vi "NormaliseProfile.vi"(5 "ResampleHeights":dbl[](array[numeric])=[25.4, 38.1, 50.8, 76.2, 101.6, 127.0, 152.4, 203.2, 254.0, 304.8, 406.4, 508.0, 609.6, 812.8, 1219.2, 1524.0], 6 "Zref":dbl=508.0 min=0.0, 7 "ResampleToN":i32, 10 "zUClusterIn":cluster{dbl[], dbl[]}, 11 "Resampler":T1) -> (1 "U(Zref)":dbl, 2 "zUClusterNormalised":cluster{dbl[], dbl[]}, 3 "zUClusterNormalisedResampled":cluster{dbl[], dbl[]})   [LabVIEW 2014]
uses:
  Resampler.ctl
  <vilib>/Analysis/NI_AALPro.lvlib
  <vilib>/gmath/NI_Gmath.lvlib
panel:
  in  "Interpolation":i32(ring)=1 items=["nearest", "linear", "spline", "cubic Hermite", "Lagrange"]
  in  "binTolerance":dbl=10.0
  out "firstBelow":dbl
  out "firstAbove":dbl
  out "XY Graph":cluster{dbl[], dbl[]}[](graph)
  # "Fit using values at  measurement Z heights"
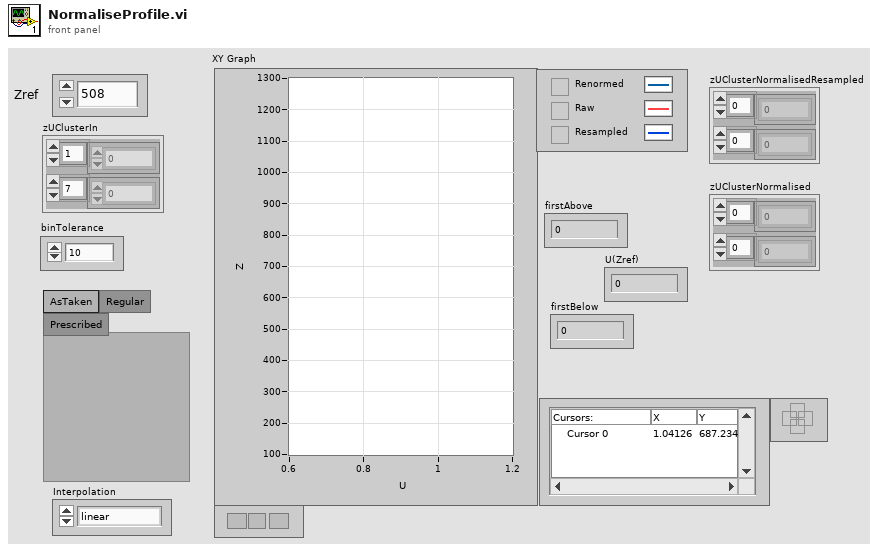
[diagram p1: front panel]
types:
  T1 = typedef "Resampler.ctl" = enum32{"AsTaken", "Regular", "Prescribed"}
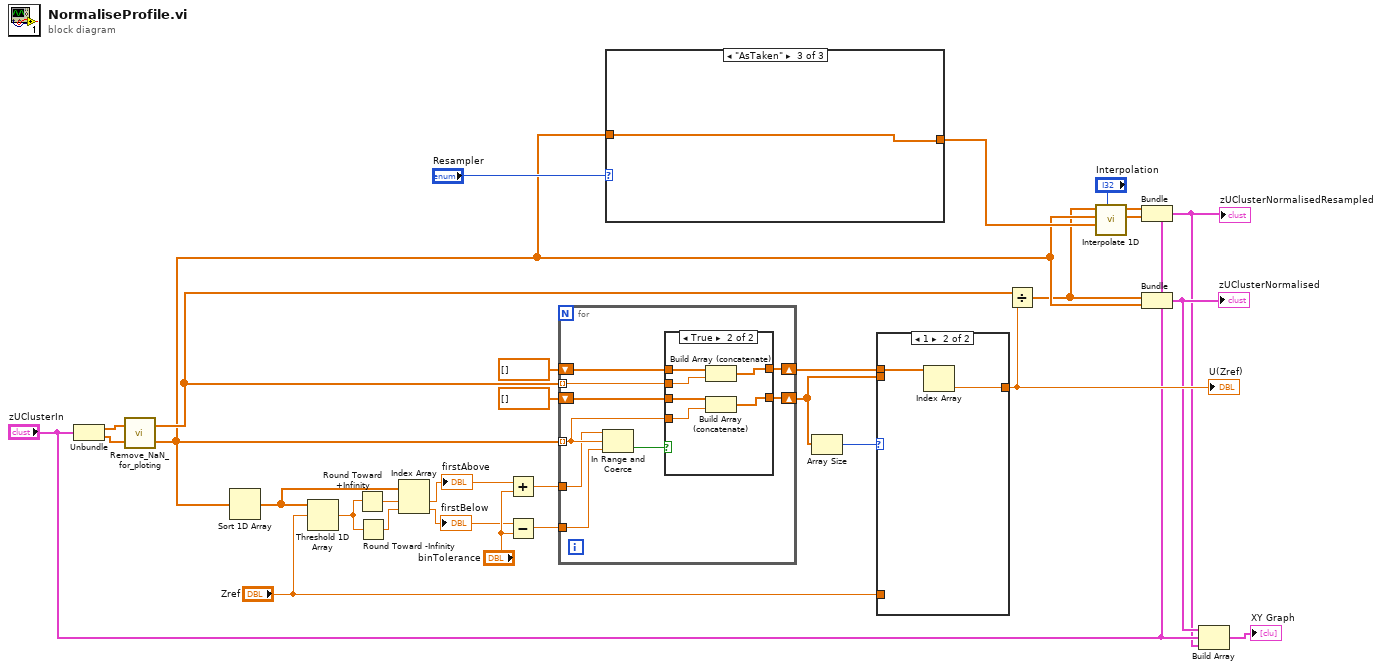
[diagram p0: block diagram]
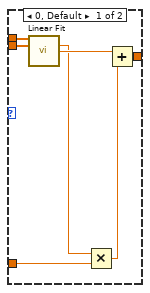
[diagram p2: hidden frame]
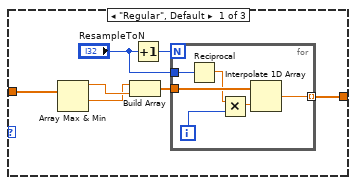
[diagram p3: hidden frame]
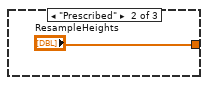
[diagram p4: hidden frame]
diagram:
  n1 = Unbundle("zUClusterIn") -> (w15:dbl[], w16:dbl[])
  n2 = call "Remove_NaN_for_ploting.vi"("Array 2"=w16, "Array 1"=w15) -> ("Array 2 Out"=w6:dbl[], "Array 1 Out"=w14:dbl[])
  n3 = Sort 1D Array(array=w6) -> (sorted array=w29:dbl[])
  n4 = Threshold 1D Array(2:"Zref", 3:w29) -> (0:w30:dbl)  [unwired: 1 in]
  n5 = Round Toward +Infinity(x=w30) -> (ceil(x): smallest int >= x=w28:dbl)
  n6 = Round Toward -Infinity(1:w30) -> (0:w27:dbl)
  n7 = Index Array(array=w29, index #1=w28, index #2=w27) -> (element #1=w4:dbl, element #2=w3:dbl)
  "firstAbove" <- w4
  "firstBelow" <- w3
  n8 = Add(x=w4, y="binTolerance") -> (x+y=w25:dbl)
  n9 = Subtract(x=w3, y="binTolerance") -> (x-y=w24:dbl)
  n10 = for {
    tunnel: w14 -> [w38] mode=indexing
    tunnel: w6 -> [w39] mode=indexing
    tunnel: w25 -> [w33]
    tunnel: w24 -> [w32]
    shift-right: [w37] -> w23
    shift-left: dbl[] [] -> [w36]
    shift-right: [w34] -> w2
    shift-left: dbl[] [] -> [w35]
    n11 = In Range and Coerce(upper limit=w33, x=w39, lower limit=w32) -> (In Range?=w31:bool)  [unwired: 1 out]
    n12 = case shown="True" w31 {
      tunnel: w39 -> [_ w47]
      tunnel: w38 -> [_ w46]
      tunnel: [w41 w45] -> w37
      tunnel: w36 -> [w41 w44]
      tunnel: w35 -> [w40 w43]
      tunnel: [w40 w42] -> w34
      frame False {
      }
      frame True {
        n13 = Build Array (concatenate)(w44, w46) -> (w45:dbl[])
        n14 = Build Array (concatenate)(w43, w47) -> (w42:dbl[])
      }
    }
  }
  n15 = case shown="\"AsTaken\"" "Resampler" {
    tunnel: [w50 "ResampleHeights" w62] -> w9
    tunnel: w6 -> [w48 _ w62]
    frame "Regular", Default {
      n16 = Array Max & Min(array=w48) -> (max value=w52:dbl, min value=w51:dbl)  [unwired: 2 out]
      n17 = Build Array(w51, w52) -> (w54:dbl[])
      n18 = Increment(x="ResampleToN") -> (x+1=w49:i32)
      n19 = for {
        N: w49 -> [_]
        tunnel: w54 -> [w60]
        tunnel: "ResampleToN" -> [w59]
        tunnel: [w56] -> w50 mode=indexing
        i -> [w55]
        n20 = Reciprocal(x=w59) -> (1/x=w57:dbl)
        n21 = Multiply(x=w57, y=w55) -> (x*y=w58:dbl)
        n22 = Interpolate 1D Array(1:w58, 2:w60) -> (0:w56:dbl)
      }
    }
    frame "Prescribed" {
    }
    frame "AsTaken" {
    }
  }
  n23 = Array Size(array=w2) -> (size(s)=w1:i32)
  n24 = case shown="1" w1 {
    tunnel: w23 -> [w69 w71]
    tunnel: "Zref" -> [w66 _]
    tunnel: [w64 w70] -> w21
    tunnel: w2 -> [w63 _]
    frame 0, Default {
      n25 = call <vilib>:"Linear Fit.vi"("Y"=w69, "X"=w63) -> ("slope"=w67:dbl, "intercept"=w68:dbl)  [unwired: 9 in, 3 out]
      n26 = Multiply(x=w67, y=w66) -> (x*y=w65:dbl)
      n27 = Add(x=w68, y=w65) -> (x+y=w64:dbl)
    }
    frame 1 {
      n28 = Index Array(array=w71) -> (element=w70:dbl)  [unwired: 1 in]
    }
  }
  "U(Zref)" <- w21
  n29 = Divide(x=w14, y=w21) -> (x/y=w5:dbl[])
  n30 = call <vilib>:"Interpolate 1D.vi"("method"="Interpolation", "xi"=w9, "X"=w6, "Y"=w5) -> ("xi used"=w11:dbl[], "yi"=w12:dbl[])  [unwired: 5 in, 1 out]
  n31 = Bundle(cluster="zUClusterIn", w12, w11) -> (w8:cluster{dbl[], dbl[]})
  "zUClusterNormalisedResampled" <- w8
  n32 = Bundle(cluster="zUClusterIn", w5, w6) -> (w19:cluster{dbl[], dbl[]})
  "zUClusterNormalised" <- w19
  n33 = Build Array(w19, "zUClusterIn", w8) -> (→"XY Graph":cluster{dbl[], dbl[]}[])
